vi "Create 2D Data Real.vi"(0 "Ampl":dbl[](array[numeric])=[0.24, 0.26, 0.35, 0.325], 2 "noise":dbl=0.003, 3 "Vsg":dbl[](array[numeric])=[0.089, 0.07933333333333334, 0.06966666666666667], 4 "width":dbl=0.003, 5 "dV":dbl=0.0001, 6 "NV":dbl=900.0, 7 "V0":dbl) -> (1 "XY Graph":cluster{dbl[], dbl[]}(graph))   [LabVIEW 2016]
uses:
  <vilib>/ptbypt/NI_PtbyPt.lvlib
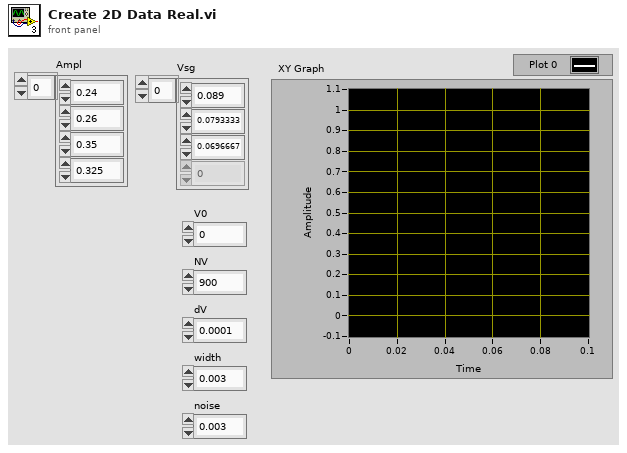
[diagram p1: front panel]
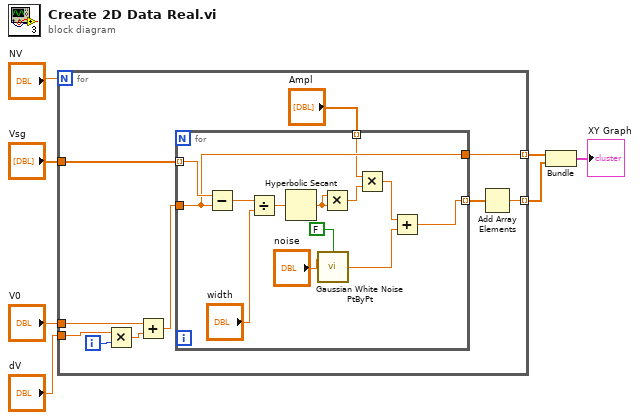
[diagram p0: block diagram]
diagram:
  n1 = for {
    N: "NV" -> [_]
    tunnel: "Vsg" -> [w17]
    tunnel: "V0" -> [w10]
    tunnel: "dV" -> [w11]
    tunnel: [w14] -> w4 mode=indexing
    tunnel: [w15] -> w3 mode=indexing
    i -> [w12]
    n2 = Multiply(x=w11, y=w12) -> (x*y=w13:dbl)
    n3 = Add(x=w10, y=w13) -> (x+y=w9:dbl)
    n4 = for {
      tunnel: w17 -> [w30] mode=indexing
      tunnel: [w21] -> w16 mode=indexing
      tunnel: [w28] -> w15
      tunnel: w9 -> [w28]
      tunnel: "Ampl" -> [w19] mode=indexing
      n5 = Subtract(x=w30, y=w28) -> (x-y=w27:dbl)
      n6 = Divide(x=w27, y="width") -> (x/y=w25:dbl)
      n7 = Hyperbolic Secant(1:w25) -> (0:w29:dbl)
      n8 = call <vilib>:"Gaussian White Noise PtByPt.vi"("initialize"=FALSE, "standard deviation"="noise") -> ("Gaussian white noise"=w24:dbl)  [unwired: 1 in]
      n9 = Multiply(x=w29, y=w29) -> (x*y=w20:dbl)
      n10 = Multiply(x=w19, y=w20) -> (x*y=w18:dbl)
      n11 = Add(x=w18, y=w24) -> (x+y=w21:dbl)
    }
    n12 = Add Array Elements(numeric array=w16) -> (sum=w14:dbl)
  }
  n13 = Bundle(w3, w4) -> (→"XY Graph":cluster{dbl[], dbl[]})  [unwired: 1 in]
